vi "ASSIGNMENT 1.vi"() -> ()   [LabVIEW 2020]
panel:
  in  "Boolean 2":bool
  out "Boolean":bool
  out "O/P":dbl
  in  "N1 2":dbl
  out "SQUARE O/P":dbl
  out "ROOT O/P":dbl
  out "DECRIMENTAL O/P":dbl
  out "INCRIMENTAL O/P":dbl
  out "Q":dbl
  out "R":dbl
  in  "SQUARE I/P":dbl
  in  "ROOT I/P":dbl
  in  "DECREMENTAL I/P":dbl
  in  "INCRIMENTAL I/P":dbl
  in  "N2":dbl
  in  "N1":dbl
  out "Divide Ans":dbl
  in  "NUM 2":dbl
  in  "NUM 1":dbl
  # "Divide"
  # "Q&R"
  # "Q&R"
  # "INCRIMENTA"
  # "DECRIMENTAL"
  # "ROOT"
  # "SQUARE"
  # "NEGELATE"
  # "BOOLEAN"
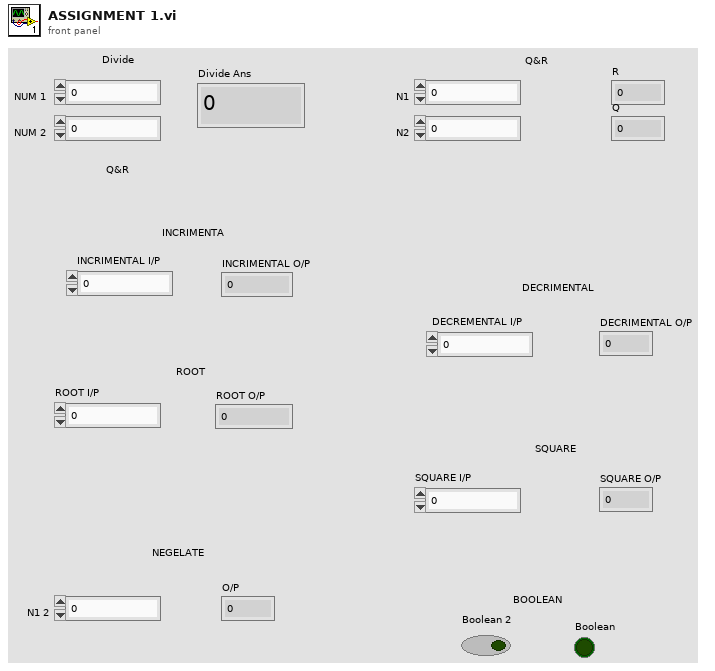
[diagram p1: front panel]
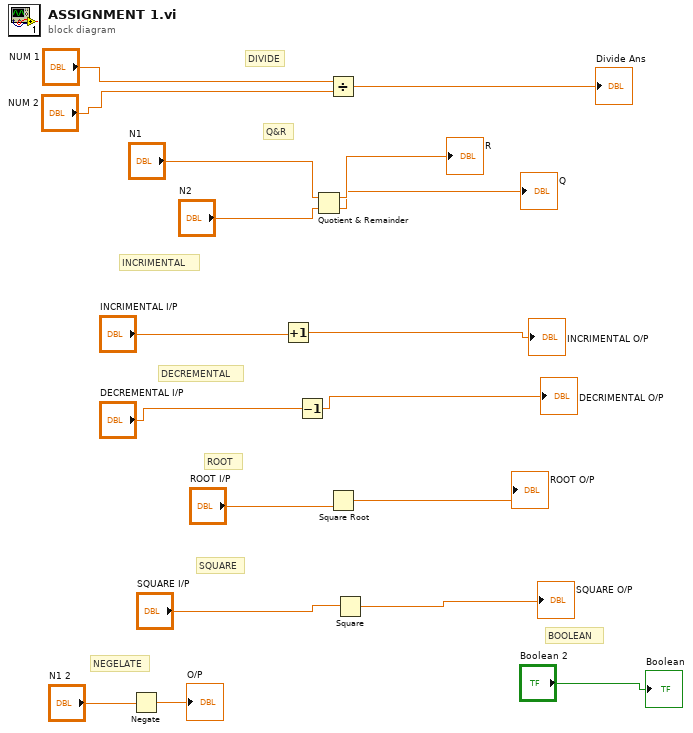
[diagram p0: block diagram]
diagram:
  # "BOOLEAN"
  # "NEGELATE"
  # "SQUARE"
  # "ROOT"
  # "DECREMENTAL"
  # "INCRIMENTAL"
  # "Q&R"
  # "DIVIDE"
  n1 = Negate(x="N1 2") -> (-x=→"O/P":dbl)
  n2 = Increment(x="INCRIMENTAL I/P") -> (x+1=→"INCRIMENTAL O/P":dbl)
  n3 = Decrement(x="DECREMENTAL I/P") -> (x-1=→"DECRIMENTAL O/P":dbl)
  n4 = Quotient & Remainder(x="N1", y="N2") -> (x-y*floor(x/y)=→"R":dbl, floor(x/y)=→"Q":dbl)
  n5 = Divide(x="NUM 1", y="NUM 2") -> (x/y=→"Divide Ans":dbl)
  n6 = Square Root(x="ROOT I/P") -> (sqrt(x)=→"ROOT O/P":dbl)
  n7 = Square(x="SQUARE I/P") -> (x^2=→"SQUARE O/P":dbl)
  "Boolean" <- "Boolean 2"
